vi "attribute_read_boolean.vi"(5 "Repeated Capability":string, 7 "Attribute":T1={"Identifier"="", "Descriptive name"="", "Data Type"=enum."Integer 32", "Command"="", "Access"=2, "Range Table"="", "Read Callback"="", "Write Callback"="", "Range Callback"="", "Check Callback"="", "Rngtable Callback"="", "Coerce Callback"="", "Supported Models"="", "Instrument Options"="", "Repeated Capabilities"="", "Check Status Callback"="", "Index"=0, "Flag: OPC Wait"=FALSE, "Flag: Dont check status"=FALSE, "Flag: Cache Only"=FALSE} {"Access" items=["Read Only", "Write Only", "Read/Write"]}, 8 "error in":errorcluster, 11 "VISA resource name":refnum<visa-resource-name>) -> (0 "error out":errorcluster, 2 "boolean out":bool, 3 "VISA resource name out":refnum<visa-resource-name>)   [LabVIEW 2014, in "rszvl_rsidr_core.lvlib"]
uses:
  rszvl_rsidr_core.lvlib
  type_Attribute.ctl
  type_Attribute_Data_Type.ctl
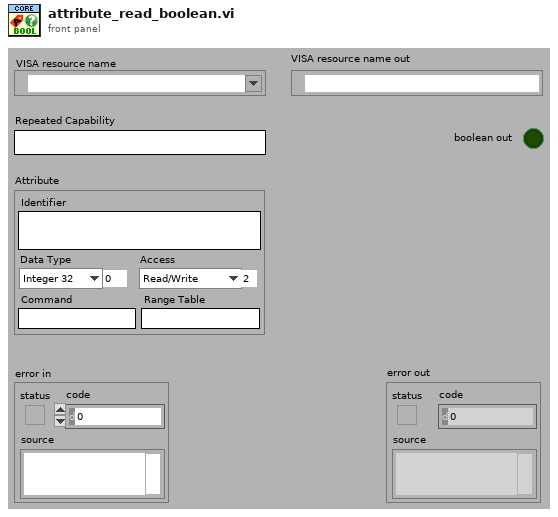
[diagram p1: front panel]
types:
  T1 = typedef "rszvl_rsidr_core.lvlib/type_Attribute.ctl" = cluster{"Identifier":string, "Descriptive name":string, "Data Type":T2, "Command":string, "Access":u16, "Range Table":string, "Read Callback":string, "Write Callback":string, "Range Callback":string, "Check Callback":string, "Rngtable Callback":string, "Coerce Callback":string, "Supported Models":string, "Instrument Options":string, "Repeated Capabilities":string, "Check Status Callback":string, "Index":i32, "Flag: OPC Wait":bool, "Flag: Dont check status":bool, "Flag: Cache Only":bool}
  T2 = typedef "rszvl_rsidr_core.lvlib/type_Attribute_Data_Type.ctl" = enum16{"Integer 32", "Double", "String", "Boolean", "None", "Integer 64"}
  T3 = typedef "rszvl_rsidr_core.lvlib/type_Session_Data.ctl" = cluster{"Instr type":string, "Instr type for err. msg.":string, "Installed Options":string[], "OPC Timeout":i32, "Query Instrument Status":bool, "Check Range":bool, "Check Options":bool, "Add LF to Write":bool, "Simulate":bool, "Logging":bool, "Logging params":variant, "Interface Type":enum16{"Unknown", "GPIB", "VXI", "GPIB_VXI", "ASRL", "PXI", "TCPIP", "USB", "SOCKET"}, "Fast Sweep":i32, "AdditionalFlags":i32, "WaitBeforeWrite":i32, "WaitBeforeRead":i32, "BinDataChunkSize":i64}
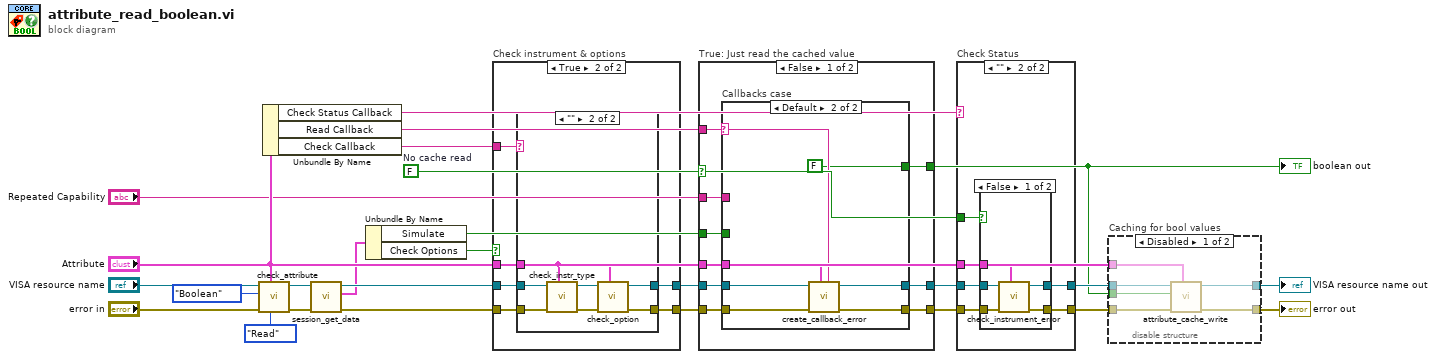
[diagram p0: block diagram]
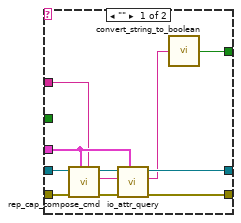
[diagram p2: hidden frame]
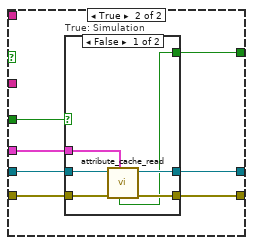
[diagram p3: hidden frame]
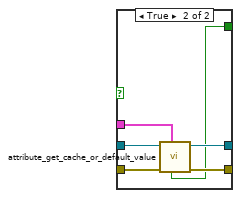
[diagram p4: hidden frame]
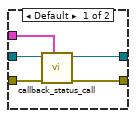
[diagram p5: hidden frame]
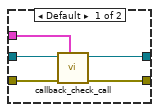
[diagram p8: hidden frame]
diagram:
  w8 = FALSE  # No cache read
  n1 = call "check_attribute.vi"("Access"=enum16{"Read", "Write"}."Read", "Attribute"="Attribute", "error in"="error in", "Data Type"=type_Attribute_Data_Type."Boolean", "VISA resource name"="VISA resource name") -> ("error out"=w13:errorcluster, "VISA resource name out"=w14:refnum<visa-resource-name>)  [unwired: 5 in]
  n2 = Unbundle By Name("Attribute") -> ("Check Status Callback"=w15:string, "Read Callback"=w16:string, "Check Callback"=w7:string)
  n3 = call "session_get_data.vi"("error in"=w13, "VISA resource name"=w14) -> ("error out"=w12:errorcluster, "Session User Data out"=w9:T3, "VISA resource name out"=w11:refnum<visa-resource-name>)  [unwired: 7 in]
  n4 = Unbundle By Name(w9) -> ("Simulate"=w2:bool, "Check Options"=w10:bool)
  n5 = case "Check instrument & options" shown="True" w10 {
    tunnel: [w28 w34] -> w5
    tunnel: [w27 w33] -> w4
    tunnel: w7 -> [_ w32]
    tunnel: w12 -> [w27 w31]
    tunnel: w11 -> [w28 w30]
    tunnel: "Attribute" -> [_ w29]
    frame False {
    }
    frame True {
      n6 = case shown="\"\"" w32 {
        tunnel: [w38 w44] -> w34
        tunnel: [w36 w43] -> w33
        tunnel: w31 -> [w37 w42]
        tunnel: w30 -> [w39 w41]
        tunnel: w29 -> [w35 w40]
        frame Default {
          n7 = call "callback_check_call.vi"("Attribute"=w35, "error in"=w37, "VISA resource name"=w39) -> ("error out"=w36:errorcluster, "VISA resource name out"=w38:refnum<visa-resource-name>)  [unwired: 7 in]
        }
        frame "" {
          n8 = call "check_instr_type.vi"("Attribute"=w40, "error in"=w42, "VISA resource name"=w41) -> ("error out"=w46:errorcluster, "VISA resource name out"=w45:refnum<visa-resource-name>)  [unwired: 6 in, 1 out]
          n9 = call "check_option.vi"("Attribute"=w40, "error in"=w46, "VISA resource name"=w45) -> ("error out"=w43:errorcluster, "VISA resource name out"=w44:refnum<visa-resource-name>)  [unwired: 7 in]
        }
      }
    }
  }
  n10 = case "True: Just read the cached value" shown="False" w8 {
    tunnel: "Repeated Capability" -> [w55 _]
    tunnel: [w54 w77] -> w17
    tunnel: [w52 w74] -> w20
    tunnel: w16 -> [w51 _]
    tunnel: w5 -> [w50 w80]
    tunnel: w4 -> [w49 w79]
    tunnel: "Attribute" -> [w48 w75]
    tunnel: w2 -> [w47 w76]
    tunnel: [w53 w78] -> w1
    frame False {
      n11 = case "Callbacks case" shown="Default" w51 {
        selector: w51 -> [_ w68]
        tunnel: w50 -> [w66 w72]
        tunnel: w49 -> [w65 w73]
        tunnel: w55 -> [w59 _]
        tunnel: [w64 w70] -> w53
        tunnel: [w58 w71] -> w54
        tunnel: [w57 FALSE ("Attribute Value Boolean")] -> w52
        tunnel: w48 -> [w60 w69]
        tunnel: w47 -> [_ _]
        frame "" {
          n12 = call "rep_cap_compose_cmd.vi"("Repeated Capability"=w59, "Attribute"=w60, "error in"=w65, "VISA resource name"=w66) -> ("error out"=w63:errorcluster, "Command out"=w62:string, "VISA resource name out"=w61:refnum<visa-resource-name>)  [unwired: 5 in]
          n13 = call "io_attr_query.vi"("Attribute"=w60, "error in"=w63, "write buffer"=w62, "VISA resource name"=w61) -> ("error out"=w58:errorcluster, "read buffer"=w56:string, "VISA resource name out"=w64:refnum<visa-resource-name>)  [unwired: 5 in]
          n14 = call "convert_string_to_boolean.vi"("String in"=w56) -> ("boolean value out"=w57:bool)  [unwired: 4 in]
        }
        frame Default {
          n15 = call "create_callback_error.vi"("Callback Name"=w68, "Attribute"=w69, "error in"=w73, "VISA resource name"=w72) -> ("error out"=w71:errorcluster, "VISA resource name out"=w70:refnum<visa-resource-name>)  [unwired: 6 in]
        }
      }
    }
    frame True {
      n16 = case "True: Simulation" shown="False" w76 {
        tunnel: w79 -> [w86 w92]
        tunnel: w80 -> [w85 w91]
        tunnel: w75 -> [w84 w88]
        tunnel: [w83 w90] -> w77
        tunnel: [w82 w89] -> w78
        tunnel: [w81 w87] -> w74
        frame False {
          n17 = call "attribute_cache_read.vi"("Attribute"=w84, "error in"=w86, "VISA resource name"=w85) -> ("error out"=w83:errorcluster, "VISA resource name out"=w82:refnum<visa-resource-name>, "Boolean out"=w81:bool)  [unwired: 1 in, 5 out]
        }
        frame True {
          n18 = call "attribute_get_cache_or_default_value.vi"("Attribute"=w88, "error in"=w92, "VISA resource name"=w91) -> ("error out"=w90:errorcluster, "VISA resource name out"=w89:refnum<visa-resource-name>, "Boolean out"=w87:bool)  [unwired: 1 in, 5 out]
        }
      }
    }
  }
  "boolean out" <- w20
  n19 = case "Check Status" shown="\"\"" w15 {
    tunnel: w17 -> [w97 w101]
    tunnel: [w96 w100] -> w25
    tunnel: [w95 w102] -> w26
    tunnel: w1 -> [w94 w103]
    tunnel: "Attribute" -> [w93 w99]
    tunnel: w8 -> [_ w98]
    frame Default {
      n20 = call "callback_status_call.vi"("Attribute"=w93, "error in"=w97, "VISA resource name"=w94) -> ("error out"=w96:errorcluster, "VISA resource name out"=w95:refnum<visa-resource-name>)  [unwired: 7 in]
    }
    frame "" {
      n21 = case shown="False" w98 {
        tunnel: w103 -> [w108 w110]
        tunnel: [w107 w110] -> w102
        tunnel: w101 -> [w106 w109]
        tunnel: [w105 w109] -> w100
        tunnel: w99 -> [w104 _]
        frame False {
          n22 = call "check_instrument_error.vi"("Attribute"=w104, "error in"=w106, "VISA resource name"=w108) -> ("error out"=w105:errorcluster, "VISA resource name out"=w107:refnum<visa-resource-name>)  [unwired: 7 in]
        }
        frame True {
        }
      }
    }
  }
  n23 = disable-structure "Caching for bool values" shown="Disabled" {
    disable-tunnel: [w116 w118] -> w19
    disable-tunnel: [w115 w117] -> w18
    disable-tunnel: w25 -> [w114 w117]
    disable-tunnel: w26 -> [w113 w118]
    disable-tunnel: w20 -> [w112 _]
    disable-tunnel: "Attribute" -> [w111 _]
    frame Disabled {
      n24 = call "attribute_cache_write.vi"("Attribute"=w111, "error in"=w114, "Value in"=w112, "VISA resource name"=w113) -> ("error out"=w115:errorcluster, "VISA resource name out"=w116:refnum<visa-resource-name>)  [unwired: 6 in]
    }
    frame Enabled {
    }
  }
  "error out" <- w18
  "VISA resource name out" <- w19
